vi "Digital_Bridge_3_kart.vi"() -> ()   [LabVIEW 2014] (continued)
                            n509 = property on="Default Values Listbox" class="LstBox (strict)"() -> ("Item Symbols"=w1275:i32[])  [unwired: 2 in, 2 out]
                            n510 = Index Array(array=w1275, index=w1268) -> (element=w1277:i32)
                            n511 = Equal?(x=w1277, y=1) -> (x = y?=w1267:bool)
                            n512 = case shown="True" w1267 {
                              frame False {
                              }
                              frame True {
                                n513 = local read "iterasyon AD"() -> (w1279:dbl)
                                n514 = Equal?(x=w1279, y=0.0) -> (x = y?=w1278:bool)
                                n515 = case shown="True" w1278 {
                                frame False {
                                }
                                frame True {
                                n516 = local read "frekans index"() -> (w1283:dbl)
                                n517 = local read "Frekanslar"() -> (w1282:dbl[])
                                n518 = local read "F Values Array"() -> (w1281:dbl[][])
                                n519 = control-ref of="Default Values Listbox"() -> (w1285:refnum<vi>)
                                n520 = Index Array(array=w1282, index=w1283) -> (element=w1284:dbl)
                                n521 = call "get_frekans_value_1D_array.vi"("LstBox Refnum"=w1285, "frekans"=w1284, "F Values Array"=w1281) -> ("output array"=w1287:dbl[])  [unwired: 7 in, 1 out]
                                n522 = for {
                                N: 20 -> [_]
                                tunnel: w1287 -> [w1292]
                                i -> [w1290]
                                n523 = Add(x=9, y=w1290) -> (x+y=w1288:i32)
                                n524 = Index Array(array=w1292, index=w1288) -> (element=w1291:dbl)
                                n525 = case shown="0, Default" w1290 {
                                tunnel: w1291 -> [w1293 w1294 w1295 w1296 w1297 w1298 w1299 w1300 w1301 w1302 w1303 w1304 w1305 w1306 w1307 w1308 w1309 w1310 w1311 w1312]
                                frame 0, Default {
                                n526 = local write "AD Xk"(w1293) -> ()
                                }
                                frame 1 {
                                n527 = local write "10R Xk"(w1294) -> ()
                                }
                                frame 2 {
                                n528 = local write "1R Xk"(w1295) -> ()
                                }
                                frame 3 {
                                n529 = local write "Wagner Xk"(w1296) -> ()
                                }
                                frame 4 {
                                n530 = local write "Kelvin Xk"(w1297) -> ()
                                }
                                frame 5 {
                                n531 = local write "AD X(k-1)"(w1298) -> ()
                                }
                                frame 6 {
                                n532 = local write "10R X(k-1)"(w1299) -> ()
                                }
                                frame 7 {
                                n533 = local write "1R X(k-1)"(w1300) -> ()
                                }
                                frame 8 {
                                n534 = local write "Wagner  X(k-1)"(w1301) -> ()
                                }
                                frame 9 {
                                n535 = local write "Kelvin X(k-1)"(w1302) -> ()
                                }
                                frame 10 {
                                n536 = local write "AD Yk"(w1303) -> ()
                                }
                                frame 11 {
                                n537 = local write "10R Yk"(w1304) -> ()
                                }
                                frame 12 {
                                n538 = local write "1R Yk"(w1305) -> ()
                                }
                                frame 13 {
                                n539 = local write "Wagner Yk"(w1306) -> ()
                                }
                                frame 14 {
                                n540 = local write "Kelvin Yk"(w1307) -> ()
                                }
                                frame 15 {
                                n541 = local write "AD Y(k-1)"(w1308) -> ()
                                }
                                frame 16 {
                                n542 = local write "10R Y(k-1)"(w1309) -> ()
                                }
                                frame 17 {
                                n543 = local write "1R Y(k-1)"(w1310) -> ()
                                }
                                frame 18 {
                                n544 = local write "Wagner Y(k-1)"(w1311) -> ()
                                }
                                frame 19 {
                                n545 = local write "Kelvin Y(k-1)"(w1312) -> ()
                                }
                                }
                                }
                                }
                                }
                              }
                            }
                          }
                        }
                      }
                      frame #3 {
                        n546 = case shown="\"Manuel\", Default" "Manuel/Otomatik" {
                          frame "Manuel", Default {
                            n547 = local read "Denge Seçimi"() -> (w1354:u8)
                            n548 = Greater?(x=w1354, y=u32 0) -> (0:w1356:bool)
                            n549 = Less?(x=w1354, y=u32 6) -> (x < y?=w1357:bool)
                            n550 = And(x=w1357, y=w1356) -> (x .and. y?=w1355:bool)
                            n551 = case shown="True" w1355 {
                              tunnel: w1354 -> [_ w1363]
                              frame False {
                                n552 = One Button Dialog(message="Manuel olarak dengeleme seçtiğiniz için\n1 ile 5 arasında bir rakam girmelisiniz\n(1. Ana denge \\ 2. 10R \\ 3. 1R \\ 4. Wagner \\ 5. Kelvin)", button name ("OK")="TAMAM") -> (true=w1361:bool)
                                n553 = case shown="True" w1361 {
                                frame False {
                                }
                                frame True {
                                }
                                }
                              }
                              frame True {
                                n554 = case shown="5" w1363 {
                                frame 1 {
                                n555 = local write "Ana denge Switch"(TRUE ("wagner switch")) -> ()
                                n556 = local write "Denge Seçimi"(u32 1 ("Çalıştırmak istediğiniz Programı Seçin")) -> ()
                                }
                                frame 2 {
                                n557 = local write "Denge Seçimi"(u32 2 ("Çalıştırmak istediğiniz Programı Seçin")) -> ()
                                n558 = local write "10R switch"(TRUE ("wagner switch")) -> ()
                                }
                                frame 3 {
                                n559 = local write "Denge Seçimi"(u32 3 ("Çalıştırmak istediğiniz Programı Seçin")) -> ()
                                n560 = local write "1R switch"(TRUE ("wagner switch")) -> ()
                                }
                                frame 4, Default {
                                n561 = local write "Denge Seçimi"(u32 4 ("Çalıştırmak istediğiniz Programı Seçin")) -> ()
                                n562 = local write "wagner switch"(TRUE ("wagner switch")) -> ()
                                }
                                frame 5 {
                                n563 = local write "Denge Seçimi"(u32 5 ("Çalıştırmak istediğiniz Programı Seçin")) -> ()
                                n564 = local write "kelvin switch"(TRUE ("wagner switch")) -> ()
                                }
                                }
                              }
                            }
                          }
                          frame "Otomatik" {
                            n565 = local write "Denge Seçimi"(u32 4 ("Çalıştırmak istediğiniz Programı Seçin")) -> ()
                            n566 = local write "wagner switch"(TRUE ("wagner switch")) -> ()
                          }
                        }
                      }
                      frame #4 {
                        n567 = local write "stop listbox"(TRUE ("stop listbox")) -> ()
                        n568 = local write "BASLAT"(FALSE ("Boolean 6")) -> ()
                      }
                      frame #5 {
                        n569 = property on="Multicolumn Listbox" class="MCListbox (strict)"("Allow Editing Cells"=FALSE) -> ()  [unwired: 2 in, 2 out]
                        n570 = local read "start time"() -> (w1382:string)
                        n571 = property on="Frekans Listbox" class="LstBox (strict)"("DisabledEnum"=T5."Disabled" ("Disabled")) -> ()  [unwired: 2 in, 2 out]
                        n572 = property on="Default Values Listbox" class="LstBox (strict)"("DisabledEnum"=T5."Disabled" ("Disabled")) -> ()  [unwired: 2 in, 2 out]
                        n573 = String Length(string=w1382) -> (length=w1384:i32)
                        n574 = Equal?(x=w1384, y=0) -> (x = y?=w1383:bool)
                        n575 = case shown="True" w1383 {
                          frame False {
                          }
                          frame True {
                            n576 = Get Date/Time In Seconds() -> (seconds since 1Jan1904=w1387:timestamp)
                            n577 = Get Date/Time String(seconds (now)=w1387, want seconds? (F)=TRUE) -> (time string=w1385:string)  [unwired: 1 in, 1 out]
                            n578 = local write "start time"(w1385) -> ()
                          }
                        }
                      }
                    }
                  }
                }
              }
            }
          }
        }
        n579 = disable-structure shown="Disabled" {
          disable-tunnel: w630 -> [w4253 _]
          disable-tunnel: w629 -> [w4252 _]
          disable-tunnel: w628 -> [w4251 _]
          disable-tunnel: [w4250 _] -> w627
          disable-tunnel: [w4249 _] -> w626
          frame Disabled {
            w4254 = FALSE  # auto start
            n580 = call-poly <vilib>:"DAQmx Write.vi"("task/channels in"=w4252, "auto start"=w4254, "data"=w4253, "error in"=w4251) -> ("task out"=w4250:refnum<k21>, "error out"=w4249:errorcluster)  [unwired: 9 in, 1 out]
          }
          frame Enabled {
          }
        }
        n581 = call-poly <vilib>:"DAQmx Write.vi"("task/channels in"=w646, "auto start"=FALSE, "data"=w643, "error in"=w644) -> ("task out"=w645:refnum<k21>, "error out"=w638:errorcluster)  [unwired: 9 in, 1 out]
        n582 = call-poly <vilib>:"DAQmx Write.vi"("task/channels in"=w651, "auto start"=FALSE, "data"=w642, "error in"=w649) -> ("task out"=w650:refnum<k21>, "error out"=w639:errorcluster)  [unwired: 9 in, 1 out]
        n583 = call-poly <vilib>:"DAQmx Write.vi"("task/channels in"=w653, "auto start"=w652, "data"=w641, "error in"=w655) -> ("task out"=w654:refnum<k21>, "error out"=w640:errorcluster)  [unwired: 9 in, 1 out]
        n584 = Compound Arithmetic op=OR(w638, w639, w640, w626, w636, w634, w632, w624, "Stop") -> (w619:bool)
        n585 = local read "Frekanslar"() -> (w607:dbl[])
        n586 = property on="Default Values Listbox" class="LstBox (strict)"() -> ("Item Names"=w610:string[])  [unwired: 2 in, 2 out]
        n587 = local read "frekans index"() -> (w608:dbl)
        n588 = Fract/Exp String To Number(string=w610) -> (number=w611:dbl[])  [unwired: 3 in, 1 out]
        n589 = Index Array(array=w607, index=w608) -> (element=w609:dbl)
        n590 = Search 1D Array(1D array=w611, element=w609, start index (0)=0) -> (index of element=w613:i32)
        n591 = for {
          N: 51 -> [_]
          i -> [w704]
          n592 = case shown="50" w704 {
            tunnel: w704 -> [w706 w711 w716 w720 w724 w733 w742 w751 w759 w769 w773 w776 w781 w784 w789 w793 w797 w801 w805 w809 w813 w817 w821 w825 w829 w832 w837 w841 w844 w852 w863 w876 w887 w899 w911 w923 w935 w947 w959 w971 w983 w995 w1007 w1019 w1031 w1043 w1055 w1067 w1079 w1094 w1116]
            frame 0, Default {
              n593 = local read "Frekanslar"() -> (w710:dbl[])
              n594 = local read "frekans index"() -> (w709:dbl)
              n595 = Index Array(array=w710, index=w709) -> (element=w705:dbl)
              n596 = local read "input values"() -> (w708:dbl[])
              n597 = Replace Array Subset(array=w708, new element=w705, index=w706) -> (w707:dbl[])
              n598 = local write "input values"(w707) -> ()
            }
            frame 1 {
              n599 = global read "DB_Global_4_kart-Test.vi" "amplitude 1/0"() -> (w712:dbl)
              n600 = local read "input values"() -> (w714:dbl[])
              n601 = Replace Array Subset(array=w714, new element=w712, index=w711) -> (w713:dbl[])
              n602 = local write "input values"(w713) -> ()
            }
            frame 2 {
              n603 = local read "Direnc 1 [ohm]"() -> (w715:dbl)
              n604 = local read "input values"() -> (w718:dbl[])
              n605 = Replace Array Subset(array=w718, new element=w715, index=w716) -> (w717:dbl[])
              n606 = local write "input values"(w717) -> ()
            }
            frame 3 {
              n607 = local read "Direnc 2 [ohm]"() -> (w719:dbl)
              n608 = local read "input values"() -> (w722:dbl[])
              n609 = Replace Array Subset(array=w722, new element=w719, index=w720) -> (w721:dbl[])
              n610 = local write "input values"(w721) -> ()
            }
            frame 4 {
              n611 = local read "Direnc 1 - Direnc 2"() -> (w731:u32)
              n612 = local read "frekans index"() -> (w727:dbl)
              n613 = local read "Frekanslar"() -> (w728:dbl[])
              n614 = Index Array(array=w728, index=w727) -> (element=w730:dbl)
              n615 = local read "AD F/P Array"() -> (w729:dbl[][])
              n616 = call "get_phase_element.vi"("index r"=w731, "hz"=w730, "Array"=w729) -> ("element"=w723:dbl)  [unwired: 8 in]
              n617 = local read "input values"() -> (w726:dbl[])
              n618 = Replace Array Subset(array=w726, new element=w723, index=w724) -> (w725:dbl[])
              n619 = local write "input values"(w725) -> ()
            }
            frame 5 {
              n620 = local read "Direnc 1 - Direnc 2"() -> (w740:u32)
              n621 = local read "frekans index"() -> (w736:dbl)
              n622 = local read "Frekanslar"() -> (w737:dbl[])
              n623 = Index Array(array=w737, index=w736) -> (element=w739:dbl)
              n624 = local read "10R F/P Array"() -> (w738:dbl[][])
              n625 = call "get_phase_element.vi"("index r"=w740, "hz"=w739, "Array"=w738) -> ("element"=w732:dbl)  [unwired: 8 in]
              n626 = local read "input values"() -> (w735:dbl[])
              n627 = Replace Array Subset(array=w735, new element=w732, index=w733) -> (w734:dbl[])
              n628 = local write "input values"(w734) -> ()
            }
            frame 6 {
              n629 = local read "Direnc 1 - Direnc 2"() -> (w749:u32)
              n630 = local read "frekans index"() -> (w745:dbl)
              n631 = local read "Frekanslar"() -> (w746:dbl[])
              n632 = Index Array(array=w746, index=w745) -> (element=w748:dbl)
              n633 = local read "1R F/P Array"() -> (w747:dbl[][])
              n634 = call "get_phase_element.vi"("index r"=w749, "hz"=w748, "Array"=w747) -> ("element"=w741:dbl)  [unwired: 8 in]
              n635 = local read "input values"() -> (w744:dbl[])
              n636 = Replace Array Subset(array=w744, new element=w741, index=w742) -> (w743:dbl[])
              n637 = local write "input values"(w743) -> ()
            }
            frame 7 {
              n638 = local read "Direnc 1 - Direnc 2"() -> (w758:u32)
              n639 = local read "frekans index"() -> (w754:dbl)
              n640 = local read "Frekanslar"() -> (w755:dbl[])
              n641 = Index Array(array=w755, index=w754) -> (element=w757:dbl)
              n642 = local read "Wagner F/P Array"() -> (w756:dbl[][])
              n643 = call "get_phase_element.vi"("index r"=w758, "hz"=w757, "Array"=w756) -> ("element"=w750:dbl)  [unwired: 8 in]
              n644 = local read "input values"() -> (w753:dbl[])
              n645 = Replace Array Subset(array=w753, new element=w750, index=w751) -> (w752:dbl[])
              n646 = local write "input values"(w752) -> ()
            }
            frame 8 {
              n647 = local read "Direnc 1 - Direnc 2"() -> (w767:u32)
              n648 = local read "frekans index"() -> (w763:dbl)
              n649 = local read "Frekanslar"() -> (w764:dbl[])
              n650 = Index Array(array=w764, index=w763) -> (element=w766:dbl)
              n651 = local read "Kelvin F/P Array"() -> (w765:dbl[][])
              n652 = call "get_phase_element.vi"("index r"=w767, "hz"=w766, "Array"=w765) -> ("element"=w760:dbl)  [unwired: 8 in]
              n653 = local read "input values"() -> (w762:dbl[])
              n654 = Replace Array Subset(array=w762, new element=w760, index=w759) -> (w761:dbl[])
              n655 = local write "input values"(w761) -> ()
            }
            frame 9 {
              n656 = local read "AD Xk"() -> (w768:dbl)
              n657 = local read "input values"() -> (w771:dbl[])
              n658 = Replace Array Subset(array=w771, new element=w768, index=w769) -> (w770:dbl[])
              n659 = local write "input values"(w770) -> ()
            }
            frame 10 {
              n660 = local read "10R Xk"() -> (w772:dbl)
              n661 = local read "input values"() -> (w775:dbl[])
              n662 = Replace Array Subset(array=w775, new element=w772, index=w773) -> (w774:dbl[])
              n663 = local write "input values"(w774) -> ()
            }
            frame 11 {
              n664 = local read "1R Xk"() -> (w777:dbl)
              n665 = local read "input values"() -> (w779:dbl[])
              n666 = Replace Array Subset(array=w779, new element=w777, index=w776) -> (w778:dbl[])
              n667 = local write "input values"(w778) -> ()
            }
            frame 12 {
              n668 = local read "Wagner Xk"() -> (w780:dbl)
              n669 = local read "input values"() -> (w783:dbl[])
              n670 = Replace Array Subset(array=w783, new element=w780, index=w781) -> (w782:dbl[])
              n671 = local write "input values"(w782) -> ()
            }
            frame 13 {
              n672 = local read "Kelvin Xk"() -> (w785:dbl)
              n673 = local read "input values"() -> (w787:dbl[])
              n674 = Replace Array Subset(array=w787, new element=w785, index=w784) -> (w786:dbl[])
              n675 = local write "input values"(w786) -> ()
            }
            frame 14 {
              n676 = local read "AD X(k-1)"() -> (w788:dbl)
              n677 = local read "input values"() -> (w791:dbl[])
              n678 = Replace Array Subset(array=w791, new element=w788, index=w789) -> (w790:dbl[])
              n679 = local write "input values"(w790) -> ()
            }
            frame 15 {
              n680 = local read "10R X(k-1)"() -> (w792:dbl)
              n681 = local read "input values"() -> (w795:dbl[])
              n682 = Replace Array Subset(array=w795, new element=w792, index=w793) -> (w794:dbl[])
              n683 = local write "input values"(w794) -> ()
            }
            frame 16 {
              n684 = local read "1R X(k-1)"() -> (w796:dbl)
              n685 = local read "input values"() -> (w799:dbl[])
              n686 = Replace Array Subset(array=w799, new element=w796, index=w797) -> (w798:dbl[])
              n687 = local write "input values"(w798) -> ()
            }
            frame 17 {
              n688 = local read "Wagner  X(k-1)"() -> (w800:dbl)
              n689 = local read "input values"() -> (w803:dbl[])
              n690 = Replace Array Subset(array=w803, new element=w800, index=w801) -> (w802:dbl[])
              n691 = local write "input values"(w802) -> ()
            }
            frame 18 {
              n692 = local read "Kelvin X(k-1)"() -> (w804:dbl)
              n693 = local read "input values"() -> (w807:dbl[])
              n694 = Replace Array Subset(array=w807, new element=w804, index=w805) -> (w806:dbl[])
              n695 = local write "input values"(w806) -> ()
            }
            frame 19 {
              n696 = local read "AD Yk"() -> (w808:dbl)
              n697 = local read "input values"() -> (w811:dbl[])
              n698 = Replace Array Subset(array=w811, new element=w808, index=w809) -> (w810:dbl[])
              n699 = local write "input values"(w810) -> ()
            }
            frame 20 {
              n700 = local read "10R Yk"() -> (w812:dbl)
              n701 = local read "input values"() -> (w815:dbl[])
              n702 = Replace Array Subset(array=w815, new element=w812, index=w813) -> (w814:dbl[])
              n703 = local write "input values"(w814) -> ()
            }
            frame 21 {
              n704 = local read "1R Yk"() -> (w816:dbl)
              n705 = local read "input values"() -> (w819:dbl[])
              n706 = Replace Array Subset(array=w819, new element=w816, index=w817) -> (w818:dbl[])
              n707 = local write "input values"(w818) -> ()
            }
            frame 22 {
              n708 = local read "Wagner Yk"() -> (w820:dbl)
              n709 = local read "input values"() -> (w823:dbl[])
              n710 = Replace Array Subset(array=w823, new element=w820, index=w821) -> (w822:dbl[])
              n711 = local write "input values"(w822) -> ()
            }
            frame 23 {
              n712 = local read "Kelvin Yk"() -> (w824:dbl)
              n713 = local read "input values"() -> (w827:dbl[])
              n714 = Replace Array Subset(array=w827, new element=w824, index=w825) -> (w826:dbl[])
              n715 = local write "input values"(w826) -> ()
            }
            frame 24 {
              n716 = local read "AD Y(k-1)"() -> (w828:dbl)
              n717 = local read "input values"() -> (w831:dbl[])
              n718 = Replace Array Subset(array=w831, new element=w828, index=w829) -> (w830:dbl[])
              n719 = local write "input values"(w830) -> ()
            }
            frame 25 {
              n720 = local read "10R Y(k-1)"() -> (w833:dbl)
              n721 = local read "input values"() -> (w835:dbl[])
              n722 = Replace Array Subset(array=w835, new element=w833, index=w832) -> (w834:dbl[])
              n723 = local write "input values"(w834) -> ()
            }
            frame 26 {
              n724 = local read "1R Y(k-1)"() -> (w836:dbl)
              n725 = local read "input values"() -> (w839:dbl[])
              n726 = Replace Array Subset(array=w839, new element=w836, index=w837) -> (w838:dbl[])
              n727 = local write "input values"(w838) -> ()
            }
            frame 27 {
              n728 = local read "Wagner Y(k-1)"() -> (w840:dbl)
              n729 = local read "input values"() -> (w843:dbl[])
              n730 = Replace Array Subset(array=w843, new element=w840, index=w841) -> (w842:dbl[])
              n731 = local write "input values"(w842) -> ()
            }
            frame 28 {
              n732 = local read "Kelvin Y(k-1)"() -> (w845:dbl)
              n733 = local read "input values"() -> (w847:dbl[])
              n734 = Replace Array Subset(array=w847, new element=w845, index=w844) -> (w846:dbl[])
              n735 = local write "input values"(w846) -> ()
            }
            frame 29 {
              n736 = local read "Output Denge Kosulu x1_x2"() -> (w857:dbl[][])
              n737 = local read "Outpu Denge Kosulu y1_y2"() -> (w856:dbl[][])
              n738 = local read "Frekanslar"() -> (w850:dbl[])
              n739 = Array Size(array=w850) -> (size(s)=w849:i32)
              n740 = local read "frekans index"() -> (w848:dbl)
              n741 = call "merge_x_y.vi"("frekans size"=w849, "y1_y2"=w856, "x1_x2"=w857) -> ("x1_x2_y1_y2"=w855:dbl[][])  [unwired: 8 in]
              n742 = Subtract(x=w852, y=29) -> (x-y=w854:i32)
              n743 = local read "input values"() -> (w859:dbl[])
              n744 = Index Array(array=w855, index (row)=w854, index (col)=w848) -> (element=w853:dbl)
              n745 = Replace Array Subset(array=w859, new element=w853, index=w852) -> (w858:dbl[])
              n746 = local write "input values"(w858) -> ()
            }
            frame 30 {
              n747 = local read "Output Denge Kosulu x1_x2"() -> (w869:dbl[][])
              n748 = local read "Outpu Denge Kosulu y1_y2"() -> (w868:dbl[][])
              n749 = local read "Frekanslar"() -> (w862:dbl[])
              n750 = Array Size(array=w862) -> (size(s)=w861:i32)
              n751 = local read "frekans index"() -> (w860:dbl)
              n752 = call "merge_x_y.vi"("frekans size"=w861, "y1_y2"=w868, "x1_x2"=w869) -> ("x1_x2_y1_y2"=w867:dbl[][])  [unwired: 8 in]
              n753 = Subtract(x=w863, y=29 ("x")) -> (x-y=w866:i32)
              n754 = local read "input values"() -> (w871:dbl[])
              n755 = Index Array(array=w867, index (row)=w866, index (col)=w860) -> (element=w865:dbl)
              n756 = Replace Array Subset(array=w871, new element=w865, index=w863) -> (w870:dbl[])
              n757 = local write "input values"(w870) -> ()
            }
            frame 31 {
              n758 = local read "Output Denge Kosulu x1_x2"() -> (w881:dbl[][])
              n759 = local read "Outpu Denge Kosulu y1_y2"() -> (w880:dbl[][])
              n760 = local read "Frekanslar"() -> (w874:dbl[])
              n761 = Array Size(array=w874) -> (size(s)=w873:i32)
              n762 = local read "frekans index"() -> (w872:dbl)
              n763 = call "merge_x_y.vi"("frekans size"=w873, "y1_y2"=w880, "x1_x2"=w881) -> ("x1_x2_y1_y2"=w879:dbl[][])  [unwired: 8 in]
              n764 = Subtract(x=w876, y=29 ("x")) -> (x-y=w878:i32)
              n765 = local read "input values"() -> (w883:dbl[])
              n766 = Index Array(array=w879, index (row)=w878, index (col)=w872) -> (element=w877:dbl)
              n767 = Replace Array Subset(array=w883, new element=w877, index=w876) -> (w882:dbl[])
              n768 = local write "input values"(w882) -> ()
            }
            frame 32 {
              n769 = local read "Output Denge Kosulu x1_x2"() -> (w893:dbl[][])
              n770 = local read "Outpu Denge Kosulu y1_y2"() -> (w892:dbl[][])
              n771 = local read "Frekanslar"() -> (w886:dbl[])
              n772 = Array Size(array=w886) -> (size(s)=w885:i32)
              n773 = local read "frekans index"() -> (w884:dbl)
              n774 = call "merge_x_y.vi"("frekans size"=w885, "y1_y2"=w892, "x1_x2"=w893) -> ("x1_x2_y1_y2"=w891:dbl[][])  [unwired: 8 in]
              n775 = Subtract(x=w887, y=29 ("x")) -> (x-y=w890:i32)
              n776 = local read "input values"() -> (w895:dbl[])
              n777 = Index Array(array=w891, index (row)=w890, index (col)=w884) -> (element=w889:dbl)
              n778 = Replace Array Subset(array=w895, new element=w889, index=w887) -> (w894:dbl[])
              n779 = local write "input values"(w894) -> ()
            }
            frame 33 {
              n780 = local read "Output Denge Kosulu x1_x2"() -> (w905:dbl[][])
              n781 = local read "Outpu Denge Kosulu y1_y2"() -> (w904:dbl[][])
              n782 = local read "Frekanslar"() -> (w898:dbl[])
              n783 = Array Size(array=w898) -> (size(s)=w897:i32)
              n784 = local read "frekans index"() -> (w896:dbl)
              n785 = call "merge_x_y.vi"("frekans size"=w897, "y1_y2"=w904, "x1_x2"=w905) -> ("x1_x2_y1_y2"=w903:dbl[][])  [unwired: 8 in]
              n786 = Subtract(x=w899, y=29 ("x")) -> (x-y=w902:i32)
              n787 = local read "input values"() -> (w907:dbl[])
              n788 = Index Array(array=w903, index (row)=w902, index (col)=w896) -> (element=w901:dbl)
              n789 = Replace Array Subset(array=w907, new element=w901, index=w899) -> (w906:dbl[])
              n790 = local write "input values"(w906) -> ()
            }
            frame 34 {
              n791 = local read "Output Denge Kosulu x1_x2"() -> (w917:dbl[][])
              n792 = local read "Outpu Denge Kosulu y1_y2"() -> (w916:dbl[][])
              n793 = local read "Frekanslar"() -> (w910:dbl[])
              n794 = Array Size(array=w910) -> (size(s)=w909:i32)
              n795 = local read "frekans index"() -> (w908:dbl)
              n796 = call "merge_x_y.vi"("frekans size"=w909, "y1_y2"=w916, "x1_x2"=w917) -> ("x1_x2_y1_y2"=w915:dbl[][])  [unwired: 8 in]
              n797 = Subtract(x=w911, y=29 ("x")) -> (x-y=w914:i32)
              n798 = local read "input values"() -> (w919:dbl[])
              n799 = Index Array(array=w915, index (row)=w914, index (col)=w908) -> (element=w913:dbl)
              n800 = Replace Array Subset(array=w919, new element=w913, index=w911) -> (w918:dbl[])
              n801 = local write "input values"(w918) -> ()
            }
            frame 35 {
              n802 = local read "Output Denge Kosulu x1_x2"() -> (w929:dbl[][])
              n803 = local read "Outpu Denge Kosulu y1_y2"() -> (w928:dbl[][])
              n804 = local read "Frekanslar"() -> (w922:dbl[])
              n805 = Array Size(array=w922) -> (size(s)=w921:i32)
              n806 = local read "frekans index"() -> (w920:dbl)
              n807 = call "merge_x_y.vi"("frekans size"=w921, "y1_y2"=w928, "x1_x2"=w929) -> ("x1_x2_y1_y2"=w927:dbl[][])  [unwired: 8 in]
              n808 = Subtract(x=w923, y=29 ("x")) -> (x-y=w926:i32)
              n809 = local read "input values"() -> (w931:dbl[])
              n810 = Index Array(array=w927, index (row)=w926, index (col)=w920) -> (element=w925:dbl)
              n811 = Replace Array Subset(array=w931, new element=w925, index=w923) -> (w930:dbl[])
              n812 = local write "input values"(w930) -> ()
            }
            frame 36 {
              n813 = local read "Output Denge Kosulu x1_x2"() -> (w941:dbl[][])
              n814 = local read "Outpu Denge Kosulu y1_y2"() -> (w940:dbl[][])
              n815 = local read "Frekanslar"() -> (w934:dbl[])
              n816 = Array Size(array=w934) -> (size(s)=w933:i32)
              n817 = local read "frekans index"() -> (w932:dbl)
              n818 = call "merge_x_y.vi"("frekans size"=w933, "y1_y2"=w940, "x1_x2"=w941) -> ("x1_x2_y1_y2"=w939:dbl[][])  [unwired: 8 in]
              n819 = Subtract(x=w935, y=29 ("x")) -> (x-y=w938:i32)
              n820 = local read "input values"() -> (w943:dbl[])
              n821 = Index Array(array=w939, index (row)=w938, index (col)=w932) -> (element=w937:dbl)
              n822 = Replace Array Subset(array=w943, new element=w937, index=w935) -> (w942:dbl[])
              n823 = local write "input values"(w942) -> ()
            }
            frame 37 {
              n824 = local read "Output Denge Kosulu x1_x2"() -> (w953:dbl[][])
              n825 = local read "Outpu Denge Kosulu y1_y2"() -> (w952:dbl[][])
              n826 = local read "Frekanslar"() -> (w946:dbl[])
              n827 = Array Size(array=w946) -> (size(s)=w945:i32)
              n828 = local read "frekans index"() -> (w944:dbl)
              n829 = call "merge_x_y.vi"("frekans size"=w945, "y1_y2"=w952, "x1_x2"=w953) -> ("x1_x2_y1_y2"=w951:dbl[][])  [unwired: 8 in]
              n830 = Subtract(x=w947, y=29 ("x")) -> (x-y=w950:i32)
              n831 = local read "input values"() -> (w955:dbl[])
              n832 = Index Array(array=w951, index (row)=w950, index (col)=w944) -> (element=w949:dbl)
              n833 = Replace Array Subset(array=w955, new element=w949, index=w947) -> (w954:dbl[])
              n834 = local write "input values"(w954) -> ()
            }
            frame 38 {
              n835 = local read "Output Denge Kosulu x1_x2"() -> (w965:dbl[][])
              n836 = local read "Outpu Denge Kosulu y1_y2"() -> (w964:dbl[][])
              n837 = local read "Frekanslar"() -> (w958:dbl[])
              n838 = Array Size(array=w958) -> (size(s)=w957:i32)
              n839 = local read "frekans index"() -> (w956:dbl)
              n840 = call "merge_x_y.vi"("frekans size"=w957, "y1_y2"=w964, "x1_x2"=w965) -> ("x1_x2_y1_y2"=w963:dbl[][])  [unwired: 8 in]
              n841 = Subtract(x=w959, y=29 ("x")) -> (x-y=w962:i32)
              n842 = local read "input values"() -> (w967:dbl[])
              n843 = Index Array(array=w963, index (row)=w962, index (col)=w956) -> (element=w961:dbl)
              n844 = Replace Array Subset(array=w967, new element=w961, index=w959) -> (w966:dbl[])
              n845 = local write "input values"(w966) -> ()
            }
            frame 39 {
              n846 = local read "Output Denge Kosulu x1_x2"() -> (w977:dbl[][])
              n847 = local read "Outpu Denge Kosulu y1_y2"() -> (w976:dbl[][])
              n848 = local read "Frekanslar"() -> (w970:dbl[])
              n849 = Array Size(array=w970) -> (size(s)=w969:i32)
              n850 = local read "frekans index"() -> (w968:dbl)
              n851 = call "merge_x_y.vi"("frekans size"=w969, "y1_y2"=w976, "x1_x2"=w977) -> ("x1_x2_y1_y2"=w975:dbl[][])  [unwired: 8 in]
              n852 = Subtract(x=w971, y=29 ("x")) -> (x-y=w974:i32)
              n853 = local read "input values"() -> (w979:dbl[])
              n854 = Index Array(array=w975, index (row)=w974, index (col)=w968) -> (element=w973:dbl)
              n855 = Replace Array Subset(array=w979, new element=w973, index=w971) -> (w978:dbl[])
              n856 = local write "input values"(w978) -> ()
            }
            frame 40 {
              n857 = local read "Output Denge Kosulu x1_x2"() -> (w989:dbl[][])
              n858 = local read "Outpu Denge Kosulu y1_y2"() -> (w988:dbl[][])
              n859 = local read "Frekanslar"() -> (w982:dbl[])
              n860 = Array Size(array=w982) -> (size(s)=w981:i32)
              n861 = local read "frekans index"() -> (w980:dbl)
              n862 = call "merge_x_y.vi"("frekans size"=w981, "y1_y2"=w988, "x1_x2"=w989) -> ("x1_x2_y1_y2"=w987:dbl[][])  [unwired: 8 in]
              n863 = Subtract(x=w983, y=29 ("x")) -> (x-y=w986:i32)
              n864 = local read "input values"() -> (w991:dbl[])
              n865 = Index Array(array=w987, index (row)=w986, index (col)=w980) -> (element=w985:dbl)
              n866 = Replace Array Subset(array=w991, new element=w985, index=w983) -> (w990:dbl[])
              n867 = local write "input values"(w990) -> ()
            }
            frame 41 {
              n868 = local read "Output Denge Kosulu x1_x2"() -> (w1001:dbl[][])
              n869 = local read "Outpu Denge Kosulu y1_y2"() -> (w1000:dbl[][])
              n870 = local read "Frekanslar"() -> (w994:dbl[])
              n871 = Array Size(array=w994) -> (size(s)=w993:i32)
              n872 = local read "frekans index"() -> (w992:dbl)
              n873 = call "merge_x_y.vi"("frekans size"=w993, "y1_y2"=w1000, "x1_x2"=w1001) -> ("x1_x2_y1_y2"=w999:dbl[][])  [unwired: 8 in]
              n874 = Subtract(x=w995, y=29 ("x")) -> (x-y=w998:i32)
              n875 = local read "input values"() -> (w1003:dbl[])
              n876 = Index Array(array=w999, index (row)=w998, index (col)=w992) -> (element=w997:dbl)
              n877 = Replace Array Subset(array=w1003, new element=w997, index=w995) -> (w1002:dbl[])
              n878 = local write "input values"(w1002) -> ()
            }
            frame 42 {
              n879 = local read "Output Denge Kosulu x1_x2"() -> (w1013:dbl[][])
              n880 = local read "Outpu Denge Kosulu y1_y2"() -> (w1012:dbl[][])
              n881 = local read "Frekanslar"() -> (w1006:dbl[])
              n882 = Array Size(array=w1006) -> (size(s)=w1005:i32)
              n883 = local read "frekans index"() -> (w1004:dbl)
              n884 = call "merge_x_y.vi"("frekans size"=w1005, "y1_y2"=w1012, "x1_x2"=w1013) -> ("x1_x2_y1_y2"=w1011:dbl[][])  [unwired: 8 in]
              n885 = Subtract(x=w1007, y=29 ("x")) -> (x-y=w1010:i32)
              n886 = local read "input values"() -> (w1015:dbl[])
              n887 = Index Array(array=w1011, index (row)=w1010, index (col)=w1004) -> (element=w1009:dbl)
              n888 = Replace Array Subset(array=w1015, new element=w1009, index=w1007) -> (w1014:dbl[])
              n889 = local write "input values"(w1014) -> ()
            }
            frame 43 {
              n890 = local read "Output Denge Kosulu x1_x2"() -> (w1025:dbl[][])
              n891 = local read "Outpu Denge Kosulu y1_y2"() -> (w1024:dbl[][])
              n892 = local read "Frekanslar"() -> (w1018:dbl[])
              n893 = Array Size(array=w1018) -> (size(s)=w1017:i32)
              n894 = local read "frekans index"() -> (w1016:dbl)
              n895 = call "merge_x_y.vi"("frekans size"=w1017, "y1_y2"=w1024, "x1_x2"=w1025) -> ("x1_x2_y1_y2"=w1023:dbl[][])  [unwired: 8 in]
              n896 = Subtract(x=w1019, y=29 ("x")) -> (x-y=w1022:i32)
              n897 = local read "input values"() -> (w1027:dbl[])
              n898 = Index Array(array=w1023, index (row)=w1022, index (col)=w1016) -> (element=w1021:dbl)
              n899 = Replace Array Subset(array=w1027, new element=w1021, index=w1019) -> (w1026:dbl[])
              n900 = local write "input values"(w1026) -> ()
            }
            frame 44 {
              n901 = local read "Output Denge Kosulu x1_x2"() -> (w1037:dbl[][])
              n902 = local read "Outpu Denge Kosulu y1_y2"() -> (w1036:dbl[][])
              n903 = local read "Frekanslar"() -> (w1030:dbl[])
              n904 = local read "frekans index"() -> (w1028:dbl)
              n905 = Array Size(array=w1030) -> (size(s)=w1029:i32)
              n906 = call "merge_x_y.vi"("frekans size"=w1029, "y1_y2"=w1036, "x1_x2"=w1037) -> ("x1_x2_y1_y2"=w1035:dbl[][])  [unwired: 8 in]
              n907 = Subtract(x=w1031, y=29 ("x")) -> (x-y=w1034:i32)
              n908 = local read "input values"() -> (w1039:dbl[])
              n909 = Index Array(array=w1035, index (row)=w1034, index (col)=w1028) -> (element=w1033:dbl)
              n910 = Replace Array Subset(array=w1039, new element=w1033, index=w1031) -> (w1038:dbl[])
              n911 = local write "input values"(w1038) -> ()
            }
            frame 45 {
              n912 = local read "Output Denge Kosulu x1_x2"() -> (w1049:dbl[][])
              n913 = local read "Outpu Denge Kosulu y1_y2"() -> (w1048:dbl[][])
              n914 = local read "Frekanslar"() -> (w1042:dbl[])
              n915 = Array Size(array=w1042) -> (size(s)=w1041:i32)
              n916 = local read "frekans index"() -> (w1040:dbl)
              n917 = call "merge_x_y.vi"("frekans size"=w1041, "y1_y2"=w1048, "x1_x2"=w1049) -> ("x1_x2_y1_y2"=w1047:dbl[][])  [unwired: 8 in]
              n918 = Subtract(x=w1043, y=29 ("x")) -> (x-y=w1046:i32)
              n919 = local read "input values"() -> (w1051:dbl[])
              n920 = Index Array(array=w1047, index (row)=w1046, index (col)=w1040) -> (element=w1045:dbl)
              n921 = Replace Array Subset(array=w1051, new element=w1045, index=w1043) -> (w1050:dbl[])
              n922 = local write "input values"(w1050) -> ()
            }
            frame 46 {
              n923 = local read "Output Denge Kosulu x1_x2"() -> (w1061:dbl[][])
              n924 = local read "Outpu Denge Kosulu y1_y2"() -> (w1060:dbl[][])
              n925 = local read "Frekanslar"() -> (w1054:dbl[])
              n926 = Array Size(array=w1054) -> (size(s)=w1053:i32)
              n927 = local read "frekans index"() -> (w1052:dbl)
              n928 = call "merge_x_y.vi"("frekans size"=w1053, "y1_y2"=w1060, "x1_x2"=w1061) -> ("x1_x2_y1_y2"=w1059:dbl[][])  [unwired: 8 in]
              n929 = Subtract(x=w1055, y=29 ("x")) -> (x-y=w1058:i32)
              n930 = local read "input values"() -> (w1063:dbl[])
              n931 = Index Array(array=w1059, index (row)=w1058, index (col)=w1052) -> (element=w1057:dbl)
              n932 = Replace Array Subset(array=w1063, new element=w1057, index=w1055) -> (w1062:dbl[])
              n933 = local write "input values"(w1062) -> ()
            }
            frame 47 {
              n934 = local read "Output Denge Kosulu x1_x2"() -> (w1073:dbl[][])
              n935 = local read "Outpu Denge Kosulu y1_y2"() -> (w1072:dbl[][])
              n936 = local read "Frekanslar"() -> (w1066:dbl[])
              n937 = Array Size(array=w1066) -> (size(s)=w1065:i32)
              n938 = local read "frekans index"() -> (w1064:dbl)
              n939 = call "merge_x_y.vi"("frekans size"=w1065, "y1_y2"=w1072, "x1_x2"=w1073) -> ("x1_x2_y1_y2"=w1071:dbl[][])  [unwired: 8 in]
              n940 = Subtract(x=w1067, y=29 ("x")) -> (x-y=w1070:i32)
              n941 = local read "input values"() -> (w1075:dbl[])
              n942 = Index Array(array=w1071, index (row)=w1070, index (col)=w1064) -> (element=w1069:dbl)
              n943 = Replace Array Subset(array=w1075, new element=w1069, index=w1067) -> (w1074:dbl[])
              n944 = local write "input values"(w1074) -> ()
            }
            frame 48 {
              n945 = local read "Output Denge Kosulu x1_x2"() -> (w1085:dbl[][])
              n946 = local read "Outpu Denge Kosulu y1_y2"() -> (w1084:dbl[][])
              n947 = local read "Frekanslar"() -> (w1078:dbl[])
              n948 = Array Size(array=w1078) -> (size(s)=w1077:i32)
              n949 = local read "frekans index"() -> (w1076:dbl)
              n950 = call "merge_x_y.vi"("frekans size"=w1077, "y1_y2"=w1084, "x1_x2"=w1085) -> ("x1_x2_y1_y2"=w1083:dbl[][])  [unwired: 8 in]
              n951 = Subtract(x=w1079, y=29 ("x")) -> (x-y=w1082:i32)
              n952 = local read "input values"() -> (w1087:dbl[])
              n953 = Index Array(array=w1083, index (row)=w1082, index (col)=w1076) -> (element=w1081:dbl)
              n954 = Replace Array Subset(array=w1087, new element=w1081, index=w1079) -> (w1086:dbl[])
              n955 = local write "input values"(w1086) -> ()
            }
            frame 49 {
              n956 = To Double Precision Float(number="value 10R") -> (double precision float=w1089:dbl)
              n957 = case shown="2" "Cp - 10R" {
                tunnel: w1089 -> [w1096 w1099 w1103 w1105 w1109]
                tunnel: [w1095 w1098 w1101 w1104 w1107] -> w1088
                frame 0, Default {
                  n958 = Multiply(x=1e-09, y=w1096) -> (x*y=w1095:dbl)
                }
                frame 1 {
                  n959 = Multiply(x=1e-08, y=w1099) -> (x*y=w1098:dbl)
                }
                frame 2 {
                  n960 = Multiply(x=1e-07, y=w1103) -> (x*y=w1101:dbl)
                }
                frame 3 {
                  n961 = Multiply(x=1e-06, y=w1105) -> (x*y=w1104:dbl)
                }
                frame 4 {
                  n962 = Multiply(x=1e-05, y=w1109) -> (x*y=w1107:dbl)
                }
              }
              n963 = local read "input values"() -> (w1090:dbl[])
              n964 = Replace Array Subset(array=w1090, new element=w1088, index=w1094) -> (w1091:dbl[])
              n965 = local write "input values"(w1091) -> ()
            }
            frame 50 {
              n966 = To Double Precision Float(number="value 1R") -> (double precision float=w1113:dbl)
              n967 = case shown="0, Default" "Cp - 1R" {
                tunnel: w1113 -> [w1118 w1121 w1125 w1127 w1131]
                tunnel: [w1117 w1120 w1123 w1126 w1129] -> w1112
                frame 0, Default {
                  n968 = Multiply(x=1e-09, y=w1118) -> (x*y=w1117:dbl)
                }
                frame 1 {
                  n969 = Multiply(x=1e-08, y=w1121) -> (x*y=w1120:dbl)
                }
                frame 2 {
                  n970 = Multiply(x=1e-07, y=w1125) -> (x*y=w1123:dbl)
                }
                frame 3 {
                  n971 = Multiply(x=1e-06, y=w1127) -> (x*y=w1126:dbl)
                }
                frame 4 {
                  n972 = Multiply(x=1e-05, y=w1131) -> (x*y=w1129:dbl)
                }
              }
              n973 = local read "input values"() -> (w1114:dbl[])
              n974 = Replace Array Subset(array=w1114, new element=w1112, index=w1116) -> (w1115:dbl[])
              n975 = local write "input values"(w1115) -> ()
            }
          }
        }
        n976 = property on="Default Values Listbox" class="LstBox (strict)"() -> ("Item Symbols"=w606:i32[])  [unwired: 2 in, 2 out]
        n977 = Index Array(array=w606, index=w613) -> (element=w604:i32)
        n978 = Equal?(x=w604, y=1) -> (x = y?=w603:bool)
        n979 = case shown="False" w603 {
          frame False {
            n980 = control-ref of="Multicolumn Listbox"() -> (w1393:refnum<vi>)
            n981 = local read "Denge Kosulu x2_y2"() -> (w1394:dbl[][])
            n982 = local read "Denge Kosulu x1_x2"() -> (w1395:dbl[][])
            n983 = local read "Denge Kosulu y1_y2"() -> (w1396:dbl[][])
            n984 = control-ref of="Frekans Listbox"() -> (w1392:refnum<vi>)
            n985 = local read "Frekanslar"() -> (w1391:dbl[])
            n986 = local read "frekans index"() -> (w1397:dbl)
            n987 = call "multicolumn.vi"("LstBox Refnum"=w1392, "Frekanslar"=w1391, "MCListbox Refnum"=w1393, "Denge Kosulu x2_y2"=w1394, "Denge Kosulu x1_x2"=w1395, "Denge Kosulu y1_y2"=w1396, "frekans index"=w1397) -> ("Output Denge Kosulu x2_y2"=w1390:dbl[][], "Output Denge Kosulu x1_x2"=w1389:dbl[][], "Outpu Denge Kosulu y1_y2"=w1388:dbl[][])  [unwired: 6 in]
            n988 = local write "Output Denge Kosulu x2_y2"(w1390) -> ()
            n989 = local write "Denge Kosulu x1_x2"(w1389) -> ()
            n990 = local write "Output Denge Kosulu x1_x2"(w1389) -> ()
            n991 = local write "Outpu Denge Kosulu y1_y2"(w1388) -> ()
            n992 = local write "Denge Kosulu y1_y2"(w1388) -> ()
            n993 = local write "Denge Kosulu x2_y2"(w1390) -> ()
          }
          frame True {
            n994 = control-ref of="Multicolumn Listbox"() -> (w1402:refnum<vi>)
            n995 = local read "Denge Kosulu x2_y2"() -> (w1403:dbl[][])
            n996 = local read "Denge Kosulu x1_x2"() -> (w1404:dbl[][])
            n997 = local read "Denge Kosulu y1_y2"() -> (w1405:dbl[][])
            n998 = control-ref of="Frekans Listbox"() -> (w1401:refnum<vi>)
            n999 = local read "Frekanslar"() -> (w1400:dbl[])
            n1000 = local read "F Values Array"() -> (w1399:dbl[][])
            n1001 = local read "frekans index"() -> (w1406:dbl)
            n1002 = call "multicolumn_pass.vi"("LstBox Refnum"=w1401, "Frekanslar"=w1400, "interrupt(F)"="interrupt", "MCListbox Refnum"=w1402, "Denge Kosulu x2_y2"=w1403, "Denge Kosulu x1_x2"=w1404, "Denge Kosulu y1_y2"=w1405, "frekans index"=w1406, "F values array"=w1399) -> ("Output Denge Kosulu x2_y2"=w1407:dbl[][], "Output Denge Kosulu x1_x2"=w1408:dbl[][], "Outpu Denge Kosulu y1_y2"=w1409:dbl[][])  [unwired: 4 in]
            n1003 = local write "Output Denge Kosulu x2_y2"(w1407) -> ()
            n1004 = local write "Output Denge Kosulu x1_x2"(w1408) -> ()
            n1005 = local write "Outpu Denge Kosulu y1_y2"(w1409) -> ()
          }
        }
        n1006 = case shown="5" "Denge Seçimi" {
          frame 1 {
            # "Bu bölümde, ilgili denge durumunun dengede olup olmadığı kontrol edilir.\n\nEğer denge sağlanmışsa, program doğrudan bir sonraki denge aşamasına geçer.\n\nAyrıca, tüm dengeler başarıyla tamamlanmış ve belirlenen ölçüm sayısına ulaşılmışsa, veriler bu alt program (subVI) aracılığıyla Excel dosyasına aktarılır."
            # "Bu bölümde, Y değerinin dengelendiği kabul edilerek, şimdi sıra X değerinin dengede olup olmadığını kontrol etmeye gelir. \n\nEğer X de dengedeyse, program bir sonraki işlem için ilgili switch case’i aktif eder. \n\nAncak Y dengede değilse, program X’i dengelemeye yönelik işlemlere yönlendirilir."
            # "Bu bölümde, X değerinin dengelendiği kabul edilerek, şimdi sıra Y değerinin dengede olup olmadığını kontrol etmeye gelir. \n\nEğer Y de dengedeyse, program bir sonraki işlem için ilgili switch case’i aktif eder. \n\nAncak Y dengede değilse, program Y’yi dengelemeye yönelik işlemlere yönlendirilir."
            # "Bu bölümde, sıfırlanacak değer cihazdan okunur. Eğer okunan değer denge koşulunu sağlıyorsa, program Kontrol Y Case’ine geçer. \n\nAncak denge koşulu sağlanmazsa, program if-else yapısına yönlendirilir ve buna göre işlem devam eder."
            # "Bu bölümde ilk olarak giriş (input) değeri sisteme uygulanır. Eğer program ilk kez çalıştırılıyorsa, global input üzerinden belirlenen ilk değer (genellikle 0 V) kullanılır. \n\nArdından, cihazdan X değerleri okunur. Bu işlem 10 kez tekrarlanır ve elde edilen ölçümlerin ortalaması alınarak bir sonuç değeri elde edilir. Bu ortalama değer, daha sonra yapılacak işlemlerde kullanılmak üzere saklanır. Özellikle, formül içinde X değerini sıfırlamak için bu bilgiye ihtiyaç duyulur. \n\nEğer girilen input değeri 8 V’tan büyükse, bu durum sistem için güvenli olmayabileceğinden program hata (error) verir ve işlemi durdurur."
            # "Bu bölümün temel amacı, ölçüm aralığını (range) artırmaktır. Program, cihazdan gelen X ve Y değerlerini okuyarak bu değerlerin belirlenen aralık içinde olup olmadığını kontrol eder. \n\nEğer değerler aralık dışındaysa, aralık tekrar artırılır ve ölçüm yeniden yapılır. \n\nAyrıca, bu süreçte input ve output değerleri global değişkenlere kaydedilir. Çünkü sonraki turda, bu kaydedilen değerler farklı bir ölçüm aralığında eğim hesaplaması için kullanılacaktır."
            # "Bu bölümde, cihaza ikinci input değeri uygulanır ve karşılık gelen output değeri okunur. Daha sonra, hem input hem de output değerleri bir formüle yerleştirilir. Bu formül sayesinde, cihazın 0’a eşitleyeceği (sıfırlayacağı) yeni bir input değeri hesaplanır ve bu değer cihaza uygulanır."
            # "Auto Phase, Read X1 Y1, Read X2 Y2, Result Phase: \n\nBu bölümler genel olarak faz ölçümü işlemini gerçekleştirir. \n\nİlk olarak, faz değeri 0’a sıfırlanır. Ardından, global input üzerinden belirlenen range (ölçüm aralığı) değeri uygulanır. Bu işlemden sonra yine global input’ta tanımlanmış olan: \n\nInput 1 verilir ve okuma yapılır (Read X1 Y1) \n\nInput 2 verilir ve okuma yapılır (Read X2 Y2) \n\nBu iki ölçüm sonucuna göre faz değeri bir formül yardımıyla hesaplanır. Elde edilen bu yeni faz değeri, ilgili F/P (frekans/faz) dizisine aktarılır. \n\nBu işlemler, sistemin doğru fazla çalışmasını sağlamak ve sonraki işlemlerde bu bilgiyi referans olarak kullanmak için gerçekleştirilir."
            # "X1 ile benzer görevi üstleniyor sadece değerler Y oluyor"
            # "X ile benzer görevi üstleniyor sadece değerler Y oluyor"
            # "IF ELSE X ile benzer görevi üstleniyor sadece değerler Y oluyor"
            # "Range Kontrol X ile benzer görevi üstleniyor sadece değerler Y oluyor"
            # "Start X ile benzer görevi üstleniyor sadece değerler Y oluyor"
            # "Reset Sens X ile benzer görevi üstleniyor sadece değerler Y oluyor"
            # "Start AD X ile benzer görevi üstleniyor sadece değerler Y oluyor"
            # "Pass subvi girmeden önce doğru range miyiz değil miyiz ölçüyor, değil ise +2 üst kademeye gidiyor"
            # "Bu bölümde, ölçüm için gerekli olan giriş (input) değerleri sisteme girilir. Girişler tamamlandıktan sonra program, ölçüm işlemini başlatmak üzere X adlı bölüme yönlendirilir. Bu adım, ölçüm sürecinin fiilen başlatıldığı ilk noktadır."
            # "Bu bölümde öncelikle, sistemin kaç kez ölçüm yaptığına işaret eden meas number (ölçüm sayısı) kontrol edilir. \nEğer bu sayı 6’dan büyükse (bu sınır kullanıcı tarafından belirlenmiştir ve değiştirilebilir), program hata verir ve reset values adlı bölüme yönlenir. Bu durum, sistemin çok fazla başarısız deneme yapmasını engellemek içindir. \nEğer ölçüm sayısı 6’dan küçükse, program global bir değişken olan sensitivity (duyarlılık) değerini ayarlar ve ardından işlemlere devam etmek üzere Start X bölümüne geçer."
            # "Bu bölümde, daha önce iterasyon (tekrarlama) yapılıp yapılmadığına bakılarak, programın hangi yöne devam edeceğine karar verilir. \n\nEğer gerekli ise, range kontrolü (ölçüm aralığının uygunluğu) yapılır veya sensitivity ayarlama (cihazın duyarlılığını belirleme) bölümlerine yönlendirilir. Bu sayede sistem, ölçüm koşullarına en uygun şekilde ayarlanarak doğru ve güvenilir sonuçlar elde edilmesi sağlanır."
            # "Bu bölümde, daha önce belirlenen F/P dizilerindeki (frekans/faz değerleri) faz bilgileri, mevcut frekansa göre uygulanır. Ardından, ilgili denge koşulunun daha önce gerçekleştirilip gerçekleştirilmediği kontrol edilir. \nEğer bu denge daha önce sağlanmamışsa, program uygun faz ayarlamasını yapar. Ancak denge daha önce zaten kurulmuşsa, faz ayarı yapılmadan işleme devam edilir. Bu sayede gereksiz tekrarların önüne geçilmiş olur."
